vi "chess_fsm.vi"() -> ()   [LabVIEW 2015]
uses:
  chess_stateinfo_cluster.ctl
  chess_piecetype_enum.ctl
  chess_teamcolor_enum.ctl
  chess_states_enum.ctl
panel:
  out "New Board Layout":cluster{"Piece Type":T1, "Team Color":T2}[][](array[cluster])
  out "Debug Dimensions":T3
  in  "stop":bool
  in  "Step":bool
  in  "Initialize":bool
  in  "Calibrate":bool
  in  "Chess State Info":T4
  out "Image Out":T6(plugin-control)
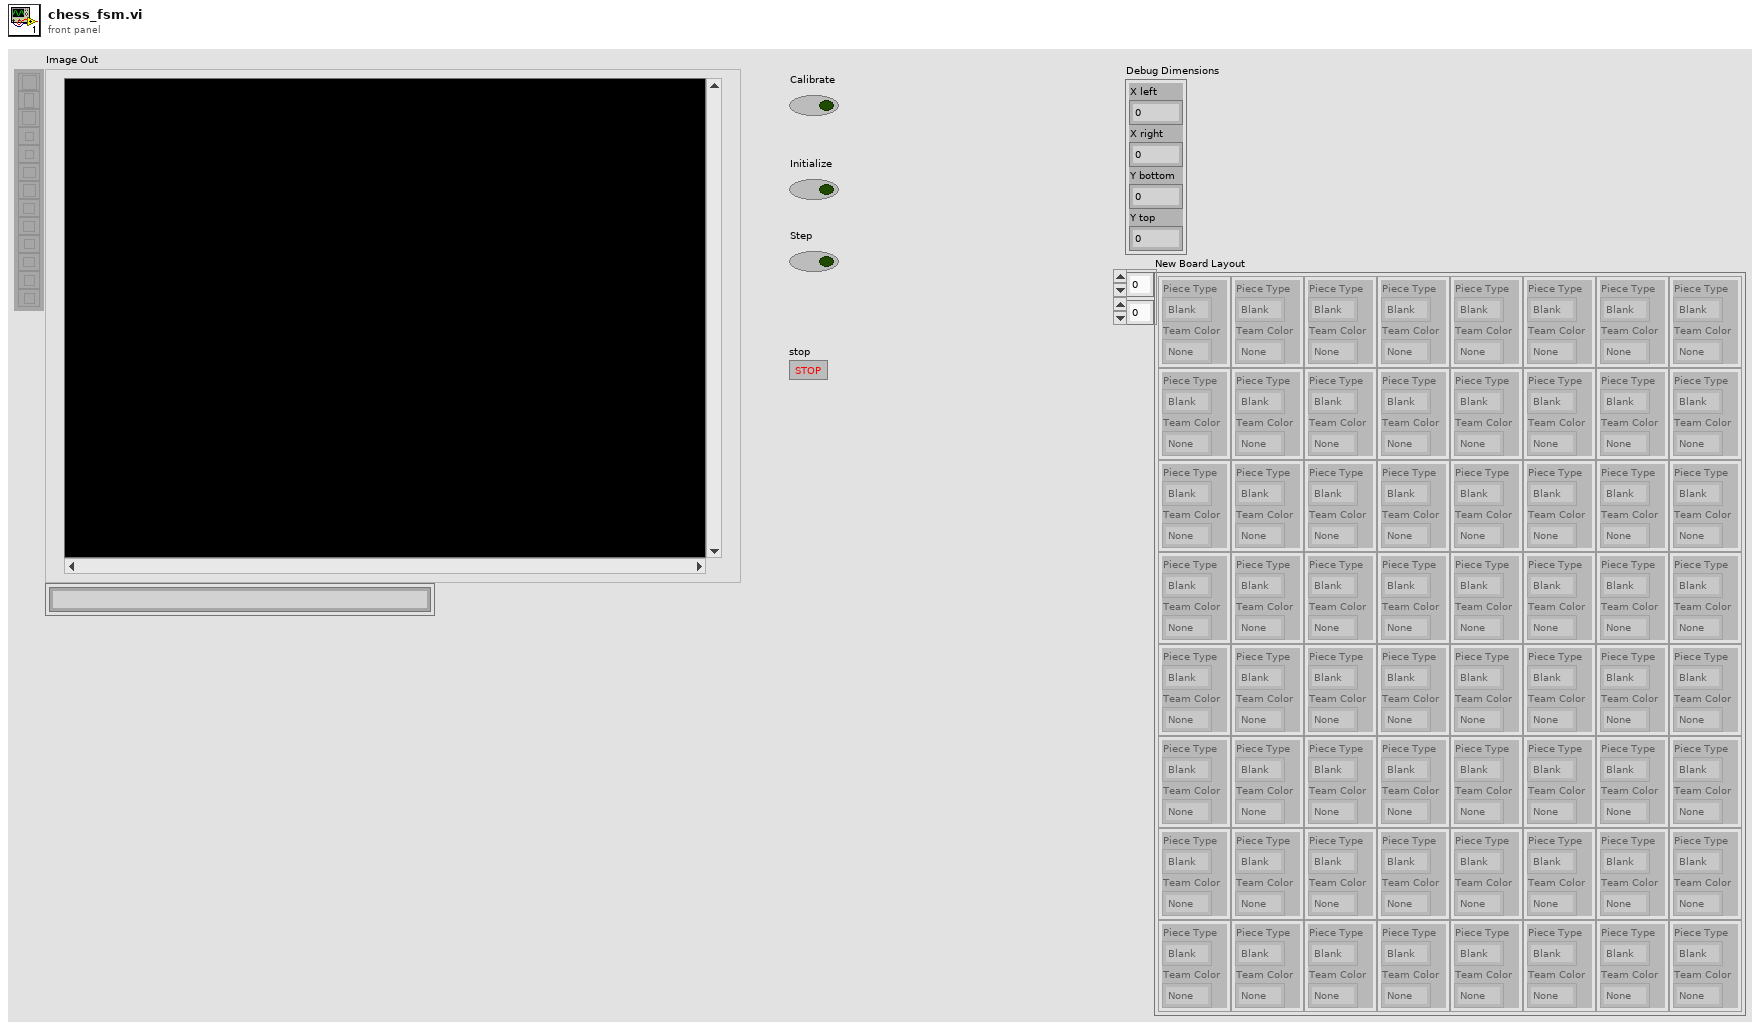
[diagram p1: front panel]
types:
  T1 = typedef "chess_piecetype_enum.ctl" = enum16{"Blank", "Pawn", "Rook", "Knight", "Bishop", "Queen", "King"}
  T2 = typedef "chess_teamcolor_enum.ctl" = enum16{"None", "Red", "Blue"}
  T3 = cluster{"X left":dbl, "X right":dbl, "Y bottom":dbl, "Y top":dbl}
  T4 = typedef "chess_stateinfo_cluster.ctl" = cluster{"Board Layout":cluster{"Piece Type":T1, "Team Color":T2}[][], "Turn":bool, "Program State":T5, "Dimensions":cluster{"X left":dbl, "X right":dbl, "Y bottom":dbl, "Y top":dbl}, "Log":string}
  T5 = typedef "chess_states_enum.ctl" = enum16{"Wait", "Calibrate", "BoardStart", "BoardStep"}
  T6 = typedef "IMAQ Image.ctl" = refnum<image>
  T7 = cluster{"Global Rectangle":cluster{"x1Left":i32, "y1Top":i32, "x2Right":i32, "y2Bottom":i32}, "Centroid":cluster{"x":sgl, "y":sgl}, "Object Size":u32, "Score":dbl}[]
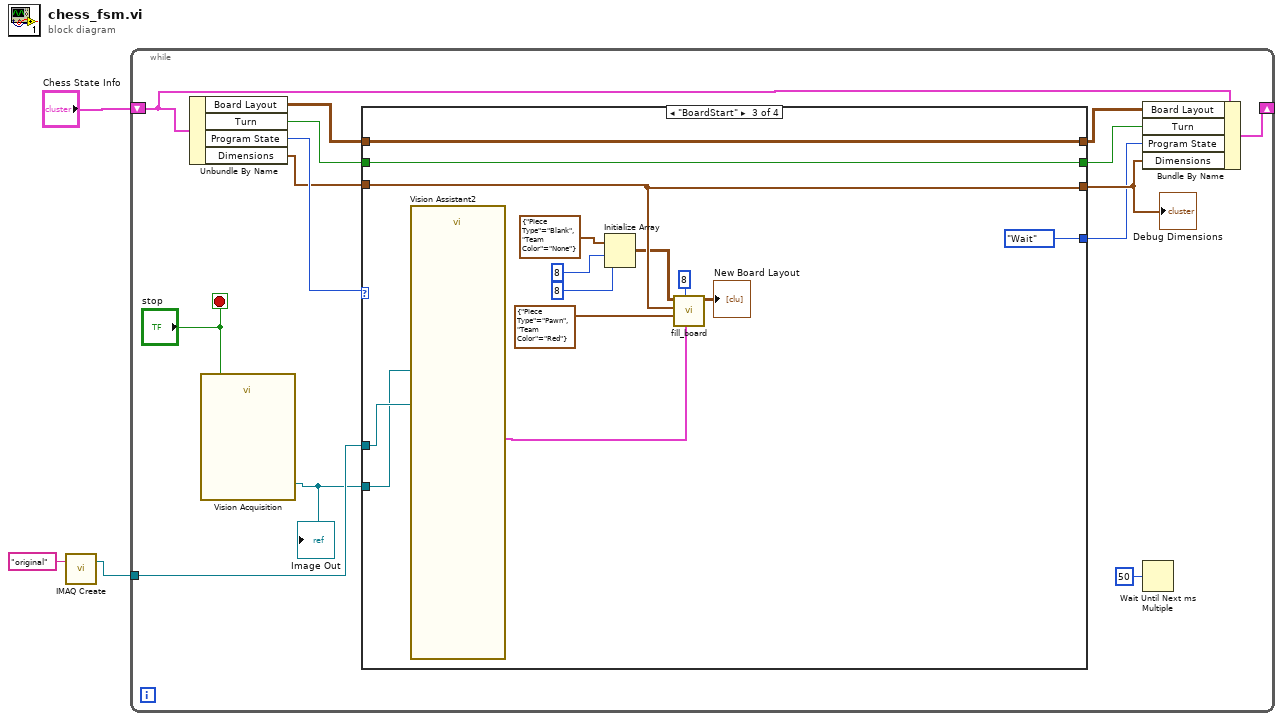
[diagram p0: block diagram]
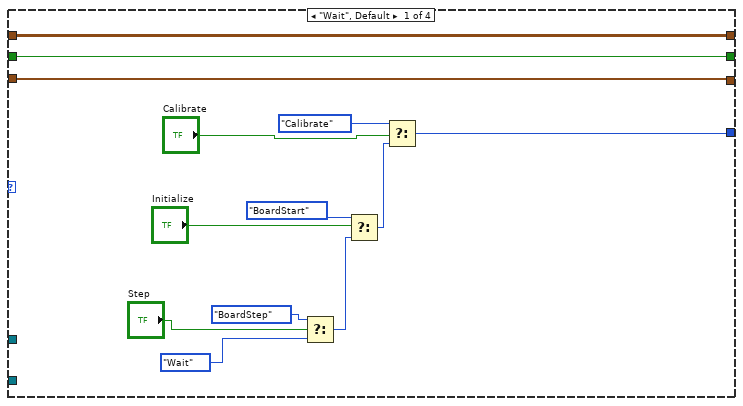
[diagram p2: hidden frame]
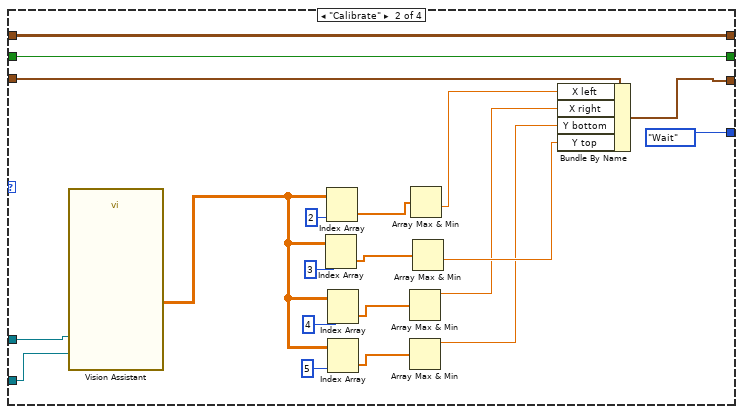
[diagram p3: hidden frame]
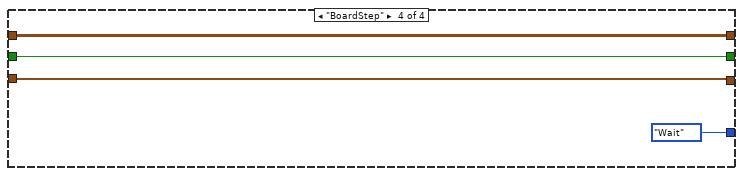
[diagram p4: hidden frame]
diagram:
  n1 = call "IMAQ Create"("Image Name"="original") -> ("New Image"=w1:T6)  [unwired: 4 in, 1 out]
  n2 = while {
    shift-right: [w14] -> _
    shift-left: "Chess State Info" -> [w13]
    tunnel: w1 -> [w6]
    stop <- "stop" stop-if-true
    n3 = Unbundle By Name(w13) -> ("Board Layout"=w15:cluster{"Piece Type":T1, "Team Color":T2}[][], "Turn"=w16:bool, "Program State"=w17:T5, "Dimensions"=w9:T3)
    n4 = call "Vision Acquisition"("Stop (F)"="stop") -> ("Image Out"=w5:T6)  [unwired: 23 in, 3 out]
    "Image Out" <- w5
    n5 = case shown="\"BoardStart\"" w17 {
      tunnel: w16 -> [w20 w49 w64 w67]
      tunnel: w15 -> [w19 w48 w55 w68]
      tunnel: [w21 chess_states_enum."Wait" ("Program State") chess_states_enum."Wait" ("Program State") chess_states_enum."Wait" ("Program State")] -> w7
      tunnel: [w20 w49 w64 w67] -> w12
      tunnel: [w19 w48 w55 w68] -> w11
      tunnel: w5 -> [_ w47 w61 _]
      tunnel: w9 -> [w18 w37 w56 w65]
      tunnel: [w18 w36 w56 w65] -> w8
      tunnel: w6 -> [_ w31 w62 _]
      frame "Wait", Default {
        n6 = Select(t=chess_states_enum."BoardStep" ("Program State"), s="Step", f=chess_states_enum."Wait" ("Program State")) -> (s? t:f=w24:T5)
        n7 = Select(t=chess_states_enum."BoardStart" ("Program State"), s="Initialize", f=w24) -> (s? t:f=w23:T5)
        n8 = Select(t=chess_states_enum."Calibrate" ("Program State"), s="Calibrate", f=w23) -> (s? t:f=w21:T5)
      }
      frame "Calibrate" {
        n9 = call "Vision Assistant"("Image In"=w47, "Image Dst"=w31) -> ("Particle Measurements (Pixels) (Particle Analysis 1)"=w45:dbl[][])  [unwired: 22 in, 3 out]
        n10 = Index Array(array=w45, index (col)=3 ("disabled index (col)")) -> (element=w40:dbl[])  [unwired: 1 in]
        n11 = Index Array(array=w45, index (col)=2 ("disabled index (col)")) -> (element=w41:dbl[])  [unwired: 1 in]
        n12 = Index Array(array=w45, index (col)=4 ("disabled index (col)")) -> (element=w39:dbl[])  [unwired: 1 in]
        n13 = Index Array(array=w45, index (col)=5 ("disabled index (col)")) -> (element=w38:dbl[])  [unwired: 1 in]
        n14 = Array Max & Min(array=w39) -> (max value=w33:dbl)  [unwired: 3 out]
        n15 = Array Max & Min(array=w38) -> (max value=w32:dbl)  [unwired: 3 out]
        n16 = Array Max & Min(array=w41) -> (min value=w35:dbl)  [unwired: 3 out]
        n17 = Array Max & Min(array=w40) -> (min value=w34:dbl)  [unwired: 3 out]
        n18 = Bundle By Name(cluster=w37, "X left"=w35, "X right"=w33, "Y bottom"=w32, "Y top"=w34) -> (w36:T3)
      }
      frame "BoardStart" {
        n19 = call "Vision Assistant2"("Image In"=w61, "Image Dst"=w62) -> ("Shape Report (Red Pawn)"=w57:T7)  [unwired: 12 in, 13 out]
        n20 = Initialize Array(cluster{"Piece Type":T1, "Team Color":T2} {"Piece Type"=enum."Blank", "Team Color"=enum."None"} ("Position State"), 8 ("dimension size"), 8 ("dimension size")) -> (w52:cluster{"Piece Type":T1, "Team Color":T2}[][])
        n21 = call "fill_board.vi"("Shape Report"=w57, "Number pieces"=8 ("Numeric"), "Replacement type"=cluster{"Piece Type":T1, "Team Color":T2} {"Piece Type"=enum."Pawn", "Team Color"=enum."Red"} ("x"), "Dimensions"=w56, "Board Layout"=w52) -> ("New Board Layout"=→"New Board Layout":cluster{"Piece Type":T1, "Team Color":T2}[][])  [unwired: 6 in]
      }
      frame "BoardStep" {
      }
    }
    "Debug Dimensions" <- w8
    n22 = Bundle By Name(cluster=w13, "Board Layout"=w11, "Turn"=w12, "Program State"=w7, "Dimensions"=w8) -> (w14:T4)
    n23 = Wait Until Next ms Multiple(millisecond multiple=u32 50) -> ()  [unwired: 1 out]
  }
